vi "Valkyrie1Buttons.vi"() -> ()   [LabVIEW 2018]
panel:
  in  "Right Trigger":bool
  in  "Left Button":bool
  in  "Right Button":bool
  out "Left":bool
  out "Right":bool
  out "Down":bool
  out "Up":bool
  out "Button X":bool
  out "Button B":bool
  out "Button A":bool
  out "Button Y":bool
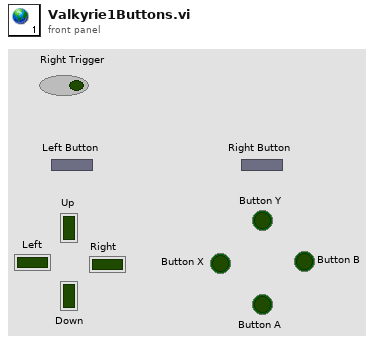
[diagram p1: front panel]
diagram:
